vi "Read Message Type.vi"(9 "Message":string) -> (1 "Ring":u16(ring) items=["None"=0, "Raw Accelerometer and Angular Rate"=193, "DeltaAngle & DeltaVelocity"=195, "Orientation Matrix"=197, "Orientation Update Matrix"=198, "Acceleration, Angular Rate & Magnetometer Vectors"=203, "Euler Angles"=206, "Temperatures"=209, "Gyro Stabilized Acceleration, Angular Rate & Magnetometer"=210])   [LabVIEW 2012, in "MicroStrain 3DM-GXx.lvlib"]
doc: "Read the message type of the input message."
uses:
  <instrlib>/MicroStrain 3DM-GXx/MicroStrain 3DM-GXx.lvlib
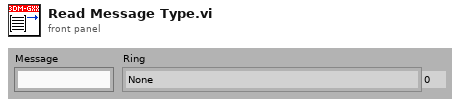
[diagram p1: front panel]
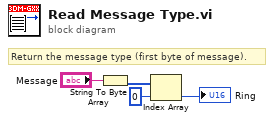
[diagram p0: block diagram]
diagram:
  # "Return the message type (first byte of message)."
  n1 = String To Byte Array(string="Message") -> (unsigned byte array=w3:u8[])
  n2 = Index Array(array=w3, index=0) -> (element=→"Ring":u8)
